vi "Generate New Data File.vi"(0 "Config":T1={"DAQ Settings"={"Trigger Type"=enum."Manual", "Trigger Samples"=0, "Pretrigger Samples"=0, "Trigger Interval"=0.0, "Time Units"=FALSE, "Auto Save"=FALSE, "Sample Rate"=7.0, "Select Analog"=FALSE, "Trigger Value"=0.0, "Trigger Stop Method"=enum."Use Samples Value to Stop Trigger", "Rate Sec/Min"=FALSE, "Save Mode"=enum."Single File", "File Size Limit"=0.0, "Log File Type"=enum."Basic", "Trigger Data Index"=0, "Log Rate"=7.0, "Rate Sec/Min (Log)"=FALSE, "Sample Rate (S/s)"=0.0, "Log Rate (S/s)"=0.0}, "Channels"=[], "Header"={"CA Number"="", "Test Name"="", "Serial Number"="", "Technician"=""}, "Graph Settings"={"Graph Labels"=[], [], [], [], [], [], [], [], [], [], [], [], [], "Graph Toggles"=[], "Axis Toggles"=[], "Graph Range"=enum."1"}, "Test Limits"=[], "All Type Info"=[], "Save Mode"=enum."Single File", "Data Base Path"=path ""} {"DAQ Settings"."Trigger Interval" min=0.0; "DAQ Settings"."Pretrigger Samples" min=0; "DAQ Settings"."Trigger Samples" min=0}, 5 "Segment File":bool, 7 "Saving Path":path, 11 "Start Time":timestamp, 12 "Base Path":path=path "C:/Data") -> (4 "new file path (Not A Path if cancelled)":path, 6 "Log Path Ref":refnum<file>)   [LabVIEW 2023]
uses:
  Type Defs and Controls/Sensor Config.ctl
  Type Defs and Controls/DAQ Settings.ctl
  Type Defs and Controls/Trigger Stop Method.ctl
  Type Defs and Controls/Log File Type.ctl
  Type Defs and Controls/Channel Config.ctl
  Type Defs and Controls/Header.ctl
  Type Defs and Controls/Graph Settings Type Def.ctl
  Type Defs and Controls/Test Limits.ctl
  Type Defs and Controls/All Part Info.ctl
  Type Defs and Controls/Part Info.ctl
panel:
  out "error out":errorcluster
  # "EGU"
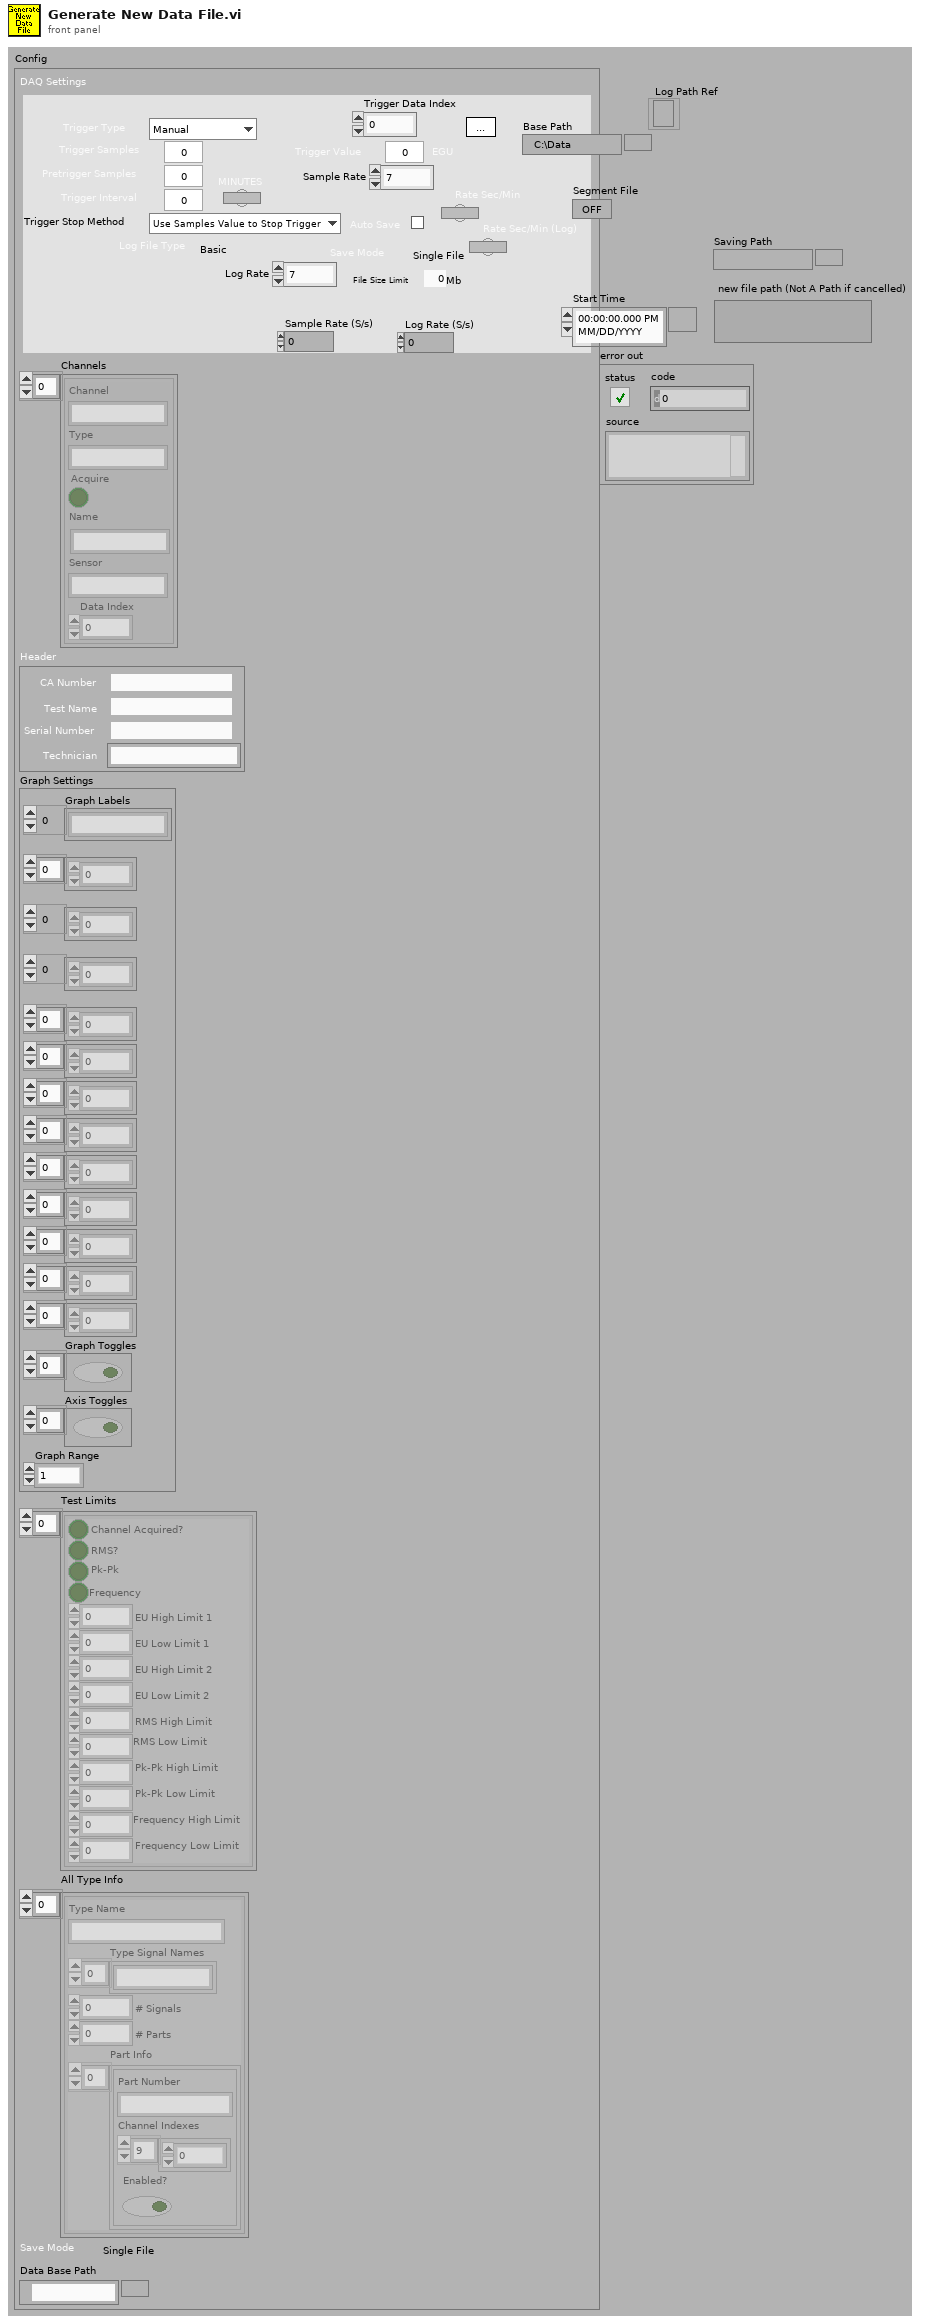
[diagram p1: front panel]
types:
  T1 = typedef "Sensor Config.ctl" = cluster{"DAQ Settings":T2, "Channels":T5[], "Header":T6, "Graph Settings":T7, "Test Limits":T8[], "All Type Info":T9, "Save Mode":enum16{"Single File", "Segmented Files", "New File at Midnight"}, "Data Base Path":path}
  T2 = typedef "DAQ Settings.ctl" = cluster{"Trigger Type":enum16{"Manual", "Timed", "Analog Rising", "Analog Falling"}, "Trigger Samples":i32, "Pretrigger Samples":i32, "Trigger Interval":dbl, "Time Units":bool, "Auto Save":bool, "Sample Rate":dbl, "Select Analog":bool, "Trigger Value":dbl, "Trigger Stop Method":T3, "Rate Sec/Min":bool, "Save Mode":enum16{"Single File", "Segmented Files", "New File at Midnight"}, "File Size Limit":dbl, "Log File Type":T4, "Trigger Data Index":u32, "Log Rate":dbl, "Rate Sec/Min (Log)":bool, "Sample Rate (S/s)":dbl, "Log Rate (S/s)":dbl}
  T3 = typedef "Trigger Stop Method.ctl" = enum16{"Use Samples Value to Stop Trigger", "Use Threshold to Stop Trigger"}
  T4 = typedef "Log File Type.ctl" = enum16{"Basic", "RTS"}
  T5 = typedef "Channel Config.ctl" = cluster{"Channel":string, "Type":string, "Acquire":bool, "Name":string, "Sensor":string, "Data Index":u32}
  T6 = typedef "Header.ctl" = cluster{"CA Number":string, "Test Name":string, "Serial Number":string, "Technician":string}
  T7 = typedef "Graph Settings Type Def.ctl" = cluster{"Graph Labels":string[], u8[], i16[], u32[], u8[], u8[], u8[], u32[], u8[], u8[], u8[], dbl[], dbl[], "Graph Toggles":bool[], "Axis Toggles":bool[], "Graph Range":enum16{"1", "2", "3", "4", "5", "10", "15", "30", "60"}}
  T8 = typedef "Test Limits.ctl" = cluster{"Channel Acquired?":bool, "RMS?":bool, "Pk-Pk":bool, "Frequency":bool, "EU High Limit 1":dbl, "EU Low Limit 1":dbl, "EU High Limit 2":dbl, "EU Low Limit 2":dbl, "RMS High Limit":dbl, "RMS Low Limit":dbl, "Pk-Pk High Limit ":dbl, "Pk-Pk Low Limit":dbl, "Frequency High Limit":dbl, "Frequency Low Limit":dbl}
  T9 = typedef "All Part Info.ctl" = cluster{"Type Name":string, "Type Signal Names":string[], "# Signals":i32, "# Parts":i32, "Part Info":T10[]}[]
  T10 = typedef "Part Info.ctl" = cluster{"Part Number":string, "Channel Indexes":u16[], "Enabled?":bool}
  T11 = enum16{"open", "replace", "create", "open or create", "replace or create", "replace or create with confirmation"}
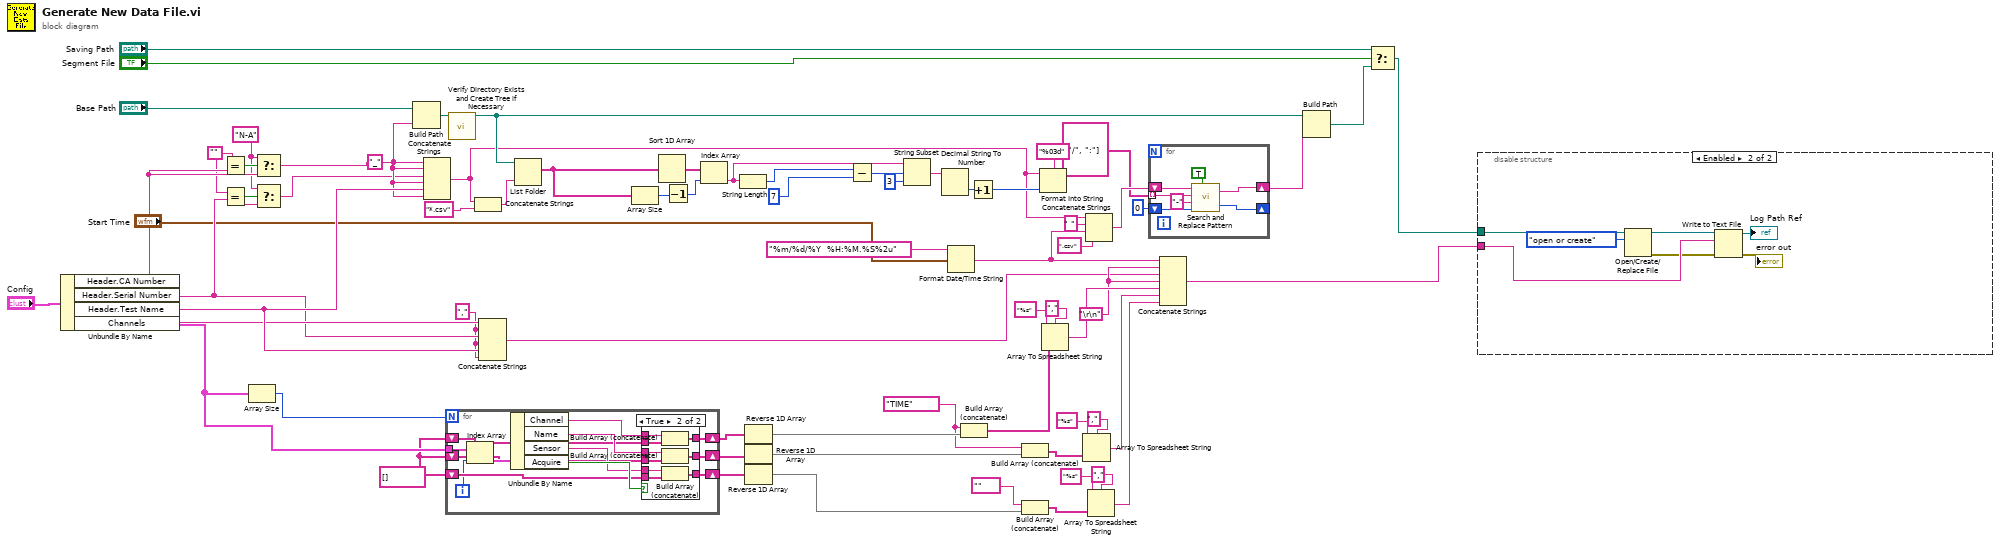
[diagram p0: block diagram]
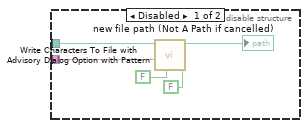
[diagram p2: hidden frame]
diagram:
  w28 = "N-A"
  w29 = ""
  w34 = "," ("string")
  w4 = "TIME" ("string")
  w35 = "\r\n"
  w5 = string[] []
  w55 = "_" ("string")
  n1 = Unbundle By Name("Config") -> ("Header.CA Number"=w68:string, "Header.Serial Number"=w67:string, "Header.Test Name"=w69:string, "Channels"=w59:T5[])
  n2 = Equal?(x=w29, y=w68) -> (x = y?=w32:bool)
  n3 = Equal?(x=w29, y=w67) -> (x = y?=w30:bool)
  n4 = Array Size(array=w59) -> (size(s)=w3:i32)
  n5 = Select(t=w28, s=w32, f=w68) -> (s? t:f=w31:string)
  n6 = Select(t=w28, s=w30, f=w67) -> (s? t:f=w27:string)
  n7 = Build Path(base path="Base Path", name or relative path=w31) -> (appended path=w56:path)
  n8 = Concatenate Strings(w31, w55, w27, w55, w69, w55) -> (w21:string)
  n9 = for {
    N: w3 -> [_]
    tunnel: w59 -> [w81]
    shift-right: [w82] -> w38
    shift-left: w5 -> [w80]
    shift-right: [w77] -> w18
    shift-left: w5 -> [w73]
    shift-right: [w72] -> w19
    shift-left: w5 -> [w71]
    i -> [w78]
    n10 = Index Array(array=w81, index=w78) -> (element=w79:T5)
    n11 = Unbundle By Name(w79) -> ("Channel"=w76:string, "Name"=w75:string, "Sensor"=w74:string, "Acquire"=w83:bool)
    n12 = case shown="True" w83 {
      tunnel: [w86 w95] -> w82
      tunnel: w80 -> [w86 w94]
      tunnel: w74 -> [_ w93]
      tunnel: [w85 w92] -> w77
      tunnel: w76 -> [_ w91]
      tunnel: w75 -> [_ w90]
      tunnel: w73 -> [w85 w89]
      tunnel: [w84 w88] -> w72
      tunnel: w71 -> [w84 w87]
      frame False {
      }
      frame True {
        n13 = Build Array (concatenate)(w91, w89) -> (w92:string[])
        n14 = Build Array (concatenate)(w90, w87) -> (w88:string[])
        n15 = Build Array (concatenate)(w93, w94) -> (w95:string[])
      }
    }
  }
  n16 = call "Verify Directory Exists and Create Tree if Necessary.vi"("path"=w56) -> ("dup path"=w41:path)  [unwired: 13 in, 1 out]
  n17 = Concatenate Strings(w21, "*.csv" ("string")) -> (w58:string)
  n18 = Concatenate Strings(w68, w34, w67, w34, w69, w34) -> (w33:string)
  n19 = List Folder(path=w41, pattern=w58) -> (filenames=w54:string[])  [unwired: 2 in, 3 out]
  n20 = Array Size(array=w54) -> (size(s)=w53:i32)
  n21 = Sort 1D Array(array=w54) -> (sorted array=w52:string[])
  n22 = Decrement(x=w53) -> (x-1=w51:i32)
  n23 = Index Array(array=w52, index=w51) -> (element=w50:string)
  n24 = String Length(string=w50) -> (length=w48:i32)
  n25 = Reverse 1D Array(array=w18) -> (reversed array=w17:string[])
  n26 = Reverse 1D Array(array=w19) -> (reversed array=w16:string[])
  n27 = Reverse 1D Array(array=w38) -> (reversed array=w14:string[])
  n28 = Subtract(x=w48, y=7) -> (x-y=w47:i32)
  n29 = String Subset(string=w50, offset (0)=w47, length (rest)=3 ("length (rest)")) -> (substring=w45:string)
  n30 = Decimal String To Number(string=w45) -> (number=w43:i32)  [unwired: 2 in, 1 out]
  n31 = Format Date/Time String(time format string (%c)="%m/%d/%Y  %H:%M.%S%2u", seconds (now)="Start Time") -> (date/time string=w1:string)  [unwired: 1 in]
  n32 = Build Array (concatenate)(w4, w17) -> (w36:string[])
  n33 = Increment(x=w43) -> (x+1=w42:i32)
  n34 = Build Array (concatenate)(w4, w16) -> (w9:string[])
  n35 = Build Array (concatenate)("" ("string"), w14) -> (w8:string[])
  n36 = Format Into String(format string="%03d", initial string=w21, w42) -> ()  [unwired: 1 in, 2 out]
  n37 = Array To Spreadsheet String(delimiter (Tab)=",", array=w36, 3:"%s" ("format string")) -> (spreadsheet string=w37:string)
  n38 = Array To Spreadsheet String(delimiter (Tab)=",", array=w9, 3:"%s" ("format string")) -> (spreadsheet string=w7:string)
  n39 = Concatenate Strings(w21, " " ("string"), w1, ".csv" ("string")) -> (w25:string)
  n40 = Array To Spreadsheet String(delimiter (Tab)=",", array=w8, 3:"%s" ("format string")) -> (spreadsheet string=w6:string)
  n41 = for {
    shift-right: [w96] -> w22
    shift-left: w25 -> [w101]
    shift-right: [w100] -> _
    shift-left: 0 ("offset past match") -> [w99]
    tunnel: string[] ["/", ":"] -> [w97] mode=indexing
    n42 = call <vilib>:"Search and Replace Pattern.vi"("string"=w101, "regular expression (\"\")"=w97, "replace string (\"\")"="-" ("replace string (\"\")"), "offset (0)"=w99, "replace all? (F)"=TRUE) -> ("result string"=w96:string, "offset past match"=w100:i32)
  }
  n43 = Concatenate Strings(w1, w35, w33, w35, w37, w7, w6) -> (w70:string)
  n44 = Build Path(base path=w41, name or relative path=w22) -> (appended path=w64:path)
  n45 = Select(t="Saving Path", s="Segment File", f=w64) -> (s? t:f=w63:path)
  n46 = disable-structure shown="Enabled" {
    disable-tunnel: w70 -> [w107 w112]
    disable-tunnel: w63 -> [w105 w114]
    frame Disabled {
      n47 = call "Write Characters To File with Advisory Dialog Option with Pattern.vi"("advisory dialog? (display:T)"=FALSE, "append to file? (new file:F)"=FALSE, "character string"=w107, "file path (dialog if empty)"=w105) -> ("new file path (Not A Path if cancelled)"=→"new file path (Not A Path if cancelled)":path)  [unwired: 6 in, 1 out]
    }
    frame Enabled {
      n48 = Open/Create/Replace File(file path (use dialog)=w114, operation (0:open)=T11."open or create") -> (refnum out=w113:refnum<file>, error out=w109:errorcluster)  [unwired: 4 in, 1 out]
      n49 = Write to Text File(file (use dialog)=w113, text=w112, error in=w109) -> (refnum out=→"Log Path Ref":refnum<file>, error out=→"error out":errorcluster)  [unwired: 1 in, 1 out]
    }
  }
